vi "Sync AO and DO CTRdriven.vi"() -> ()   [LabVIEW 2021]
doc: "I. Description:\nThis example demonstrates how to continuously acquire and generate data at the same time, synchronized with one another.\n\nII. Instructions for Running:\n1. Select the physical channel to correspond to where your signal is input on the DAQ device. Also, select the corresponding channel for where your signal is being generated.\n2. Enter the minimum and maximum voltage ranges.\nNote: For better accuracy try to match the input range to the expected voltage level of the measured signal.\n3. Set the sample rate of the acquisition.\nNote: The rate should be at least twice as fast as the maximum frequency component of the signal being acquired. \n6. Select the Rate for the generation\n7. Select what type of signal to generate and the amplitude.\nNote: This example requires two DMA channels to run. If your hardware does not support two DMA channels, you need to set the Data Transfer Mechanism property for the Analog Output Task to use \"Interrupts\". The Data Transfer Mechanism property is located in the DAQmx Channel Property hierarchy at:\n\nDAQmx Channel Property Node>>Analog Output>>General Properties>>Advanced>>Data Transfer and Memory>>Data Transfer Mechanism\n\nRefer to your device documentation to determine how many DMA channels are supported for your hardware.\n\nIII. Block Diagram Steps:\n1. Create an analog input voltage channel. Also, create an analog output voltage channel.\n2. Set the rate for the sample clock. Additionally, define the sample mode to be continuous. Also, set the sample clock rate for the signal generation.\n2a. Call the Get Terminal Name with Device Prefix VI. This will take a Task and a terminal and create a properly formatted device + terminal name to use as the source of the Trigger.\n3. Define the parameters for a Digital Edge Start Trigger. Set the Analog output to trigger off the AI Start Trigger. This is an internal trigger signal.\n4. Use the Basic Function Generator VI to create the signal to be generated.\n5. Call the Start VI to arm the two functions. Make sure the analog output is armed before the analog input. This will ensure both will start at the same time.\n6. Read the waveform data in a loop until the user hits the stop button or an error occurs. The Is Task Done? VI is used to check for errors in the Analog Output Task.\n7. Call the Clear VI to Clear the Task\n8. Use the popup dialog box to display an error if any.\n\nIV. I/O Connections Overview:\nMake sure your signal input/output terminals match the Physical Channel I/O controls."
uses:
  <vilib>/Utility/error.llb/DialogType.ctl
  <vilib>/DAQmx/write.llb/DAQmx Write (Analog Wfm 1Chan NSamp).vi
  <vilib>/DAQmx/write.llb/DAQmx Write (Digital Wfm 1Chan NSamp).vi
  <vilib>/DAQmx/create/channels.llb/DAQmx Create Channel (DO-Digital Output).vi
  <vilib>/DAQmx/configure/timing.llb/DAQmx Timing (Sample Clock).vi
  <vilib>/DAQmx/create/channels.llb/DAQmx Create Channel (CO-Pulse Generation-Frequency).vi
  <vilib>/DAQmx/configure/timing.llb/DAQmx Timing (Implicit).vi
  <vilib>/DAQmx/create/channels.llb/DAQmx Create Channel (AO-Voltage-Basic).vi
  <vilib>/Waveform/DWDTOps.llb/Digital Pattern Generator (Ramp).vi
  <vilib>/Waveform/DWDTOps.llb/DWDT Uncompress Digital.vi
  <vilib>/DAQmx/miscellaneous.llb/DAQmx Fill In Error Info.vi
  <vilib>/Waveform/DWDTOps.llb/DWDT Digital Signal Subset.vi
  <vilib>/Waveform/DWDTOps.llb/DWDT Invert Digital.vi
  <resource>/objmgr/daqmx.rc
panel:
  out "Waveform Graph":dynamicdata(graph)
  out "Digital Waveform Graph":digitalwaveform(graph)
  out "Actual Update Generation Rate":dbl=5000.0 format="%0.2f"
  out "Actual Input Rate":dbl=10000.0 format="%0.2f"
  in  "rate":dbl=1000.0 caption="Analog Output Update Rate" format="%0.2f"
  in  "minimum value":dbl=-10.0 caption="Output Minimum Value" format="%0.2f"
  in  "maximum value":dbl=10.0 caption="Output Maximum Value" format="%0.2f"
  in  "physical channels":tag="Dev1/ao0" caption="Analog Output Physical Channel"
  in  "Physical Channel":tag="Dev1/port0/line0" caption="Digital Output Physical Channel"
  in  "Rate":dbl=1000.0 caption="Digital Output Update Rate" format="%0.2f"
  in  "stop":bool
  # "For instructions, select Help>>Show Context Help"
  # "Output Channel Parameters"
  # "Timing Parameters"
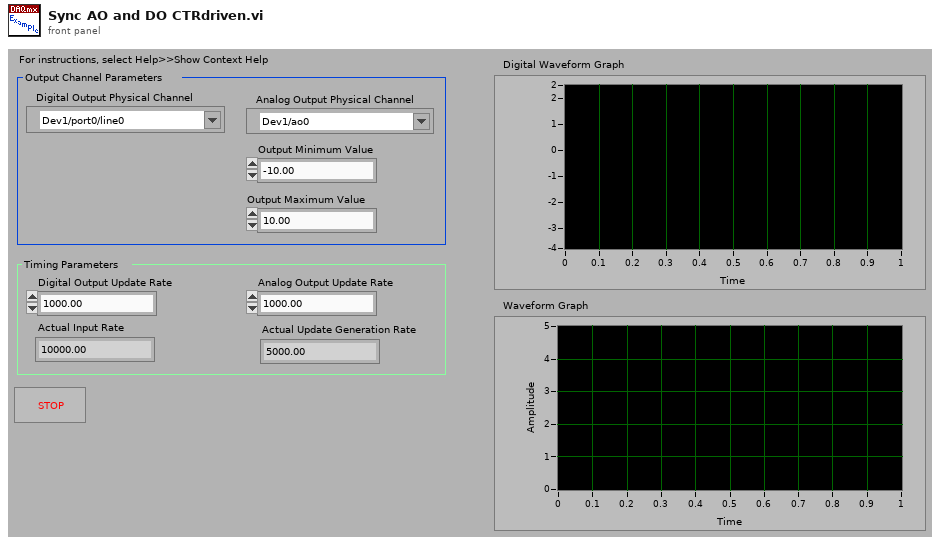
[diagram p1: front panel]
types:
  T1 = typedef "DialogType.ctl" = u16
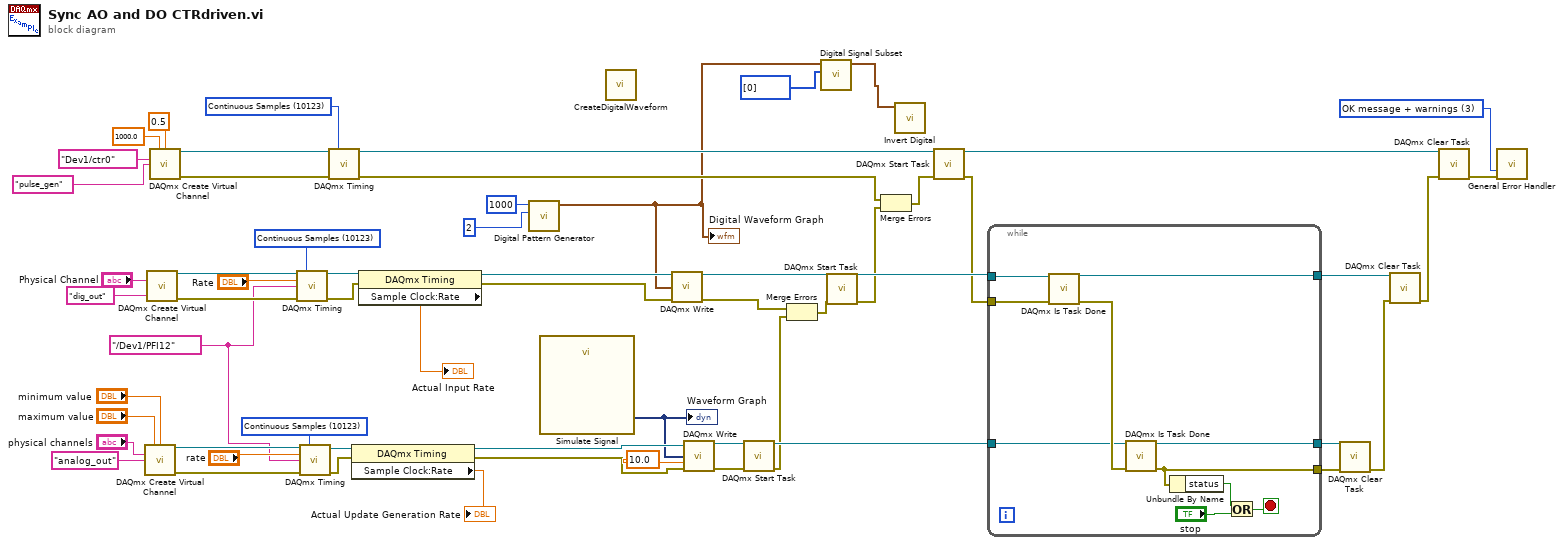
[diagram p0: block diagram]
diagram:
  w10 = 10123 items=["Finite Samples"=10178, "Continuous Samples"=10123, "Hardware Timed Single Point"=12522] ("sample mode")
  w6 = tag "/Dev1/PFI12" ("source")
  w43 = T1 3 items=["no dialog", "OK message", "continue or stop message", "OK message + warnings", "continue/stop + warnings"] ("type of dialog (OK msg:1)")
  w53 = 10123 items=["Finite Samples"=10178, "Continuous Samples"=10123] ("sample mode")
  w59 = 10123 items=["Finite Samples"=10178, "Continuous Samples"=10123] ("sample mode")
  n1 = call-poly <vilib>:"DAQmx Create Virtual Channel.vi"("maximum value"="maximum value", "minimum value"="minimum value", "physical channels"="physical channels", "name to assign"="analog_out") -> ("task out"=w52:refnum<k21>, "error out"=w51:errorcluster)  [unwired: 5 in, 5 out]
  n2 = call-poly <vilib>:"DAQmx Create Virtual Channel.vi"("lines"="Physical Channel", "name to assign"="dig_out") -> ("task out"=w57:refnum<k21>, "error out"=w58:errorcluster)  [unwired: 5 in, 7 out]
  n3 = call-poly <vilib>:"DAQmx Create Virtual Channel.vi"("frequency"=1000.0 ("High Time"), "duty cycle"=0.5 ("Low Time"), "counter"=tag "Dev1/ctr0" ("Counter(s)"), "name to assign"="pulse_gen") -> ("task out"=w12:refnum<k21>, "error out"=w11:errorcluster)  [unwired: 5 in, 5 out]
  n4 = call-poly <vilib>:"DAQmx Timing.vi"("task/channels in"=w57, "sample mode"=w59, "rate"="Rate", "source"=w6, "error in"=w58) -> ("task out"=w33:refnum<k21>, "error out"=w32:errorcluster)  [unwired: 2 in, 7 out]
  n5 = call-poly <vilib>:"DAQmx Timing.vi"("task/channels in"=w52, "sample mode"=w53, "rate"="rate", "source"=w6, "error in"=w51) -> ("task out"=w40:refnum<k21>, "error out"=w39:errorcluster)  [unwired: 2 in, 7 out]
  n6 = call-poly <vilib>:"DAQmx Timing.vi"("task/channels in"=w12, "sample mode"=w10, "error in"=w11) -> ("task out"=w9:refnum<k21>, "error out"=w8:errorcluster)  [unwired: 11 in]
  n7 = property class="DAQmx Timing"(reference=w40, error in=w39) -> (reference out=w41:refnum<k21>, error out=w38:errorcluster, "Sample Clock:Rate"=→"Actual Update Generation Rate":dbl)
  n8 = property class="DAQmx Timing"(reference=w33, error in=w32) -> (reference out=w28:refnum<k21>, error out=w27:errorcluster, "Sample Clock:Rate"=→"Actual Input Rate":dbl)
  n9 = call-poly <vilib>:"Digital Pattern Generator.vi"("number of signals"=u32 2, "number of samples"=u32 1000) -> ("digital waveform"=w1:digitalwaveform)  [unwired: 8 in, 1 out]
  "Digital Waveform Graph" <- w1
  n10 = call "Simulate Signal"() -> ("Triangle"=w24:dynamicdata)  [unwired: 6 in, 9 out]
  "Waveform Graph" <- w24
  n11 = call "CreateDigitalWaveform.vi"() -> ()  [unwired: 1 out]
  n12 = call-poly <vilib>:"DAQmx Write.vi"("task/channels in"=w28, "data"=w1, "error in"=w27) -> ("task out"=w25:refnum<k21>, "error out"=w26:errorcluster)  [unwired: 2 in, 9 out]
  n13 = call-poly <vilib>:"DAQmx Write.vi"("task/channels in"=w41, "data"=w24, "timeout"=10.0 ("Wirite Timeout"), "error in"=w38) -> ("task out"=w46:refnum<k21>, "error out"=w45:errorcluster)  [unwired: 1 in, 9 out]
  n14 = call <vilib>:"DAQmx Start Task.vi"("task/channels in"=w46, "error in"=w45) -> ("task out"=w50:refnum<k21>, "error out"=w36:errorcluster)  [unwired: 12 out]
  n15 = Merge Errors(w26, w36) -> (w35:errorcluster)
  n16 = call-poly <vilib>:"Digital Signal Subset.vi"("signals"=i32[] [0], "digital waveform"=w1) -> ("digital subset"=w2:digitalwaveform)  [unwired: 8 in, 1 out]
  n17 = call <vilib>:"DAQmx Start Task.vi"("task/channels in"=w25, "error in"=w35) -> ("task out"=w37:refnum<k21>, "error out"=w20:errorcluster)  [unwired: 12 out]
  n18 = Merge Errors(w8, w20) -> (w19:errorcluster)
  n19 = call-poly <vilib>:"Invert Digital.vi"("digital waveform"=w2) -> ()  [unwired: 9 in, 2 out]
  n20 = call <vilib>:"DAQmx Start Task.vi"("task/channels in"=w9, "error in"=w19) -> ("task out"=w17:refnum<k21>, "error out"=w18:errorcluster)  [unwired: 12 out]
  n21 = while {
    tunnel: [w70] -> w60
    tunnel: w50 -> [w65]
    tunnel: [w64] -> w49
    tunnel: w37 -> [w63]
    tunnel: w18 -> [w62]
    tunnel: [w61] -> w30
    stop <- w69 stop-if-true
    n22 = call <vilib>:"DAQmx Is Task Done.vi"("task/channels in"=w63, "error in"=w62) -> ("task out"=w70:refnum<k21>, "error out"=w66:errorcluster)  [unwired: 2 in, 10 out]
    n23 = call <vilib>:"DAQmx Is Task Done.vi"("task/channels in"=w65, "error in"=w66) -> ("task out"=w64:refnum<k21>, "error out"=w61:errorcluster)  [unwired: 12 out]
    n24 = Unbundle By Name(w61) -> ("status"=w67:bool)
    n25 = Or(x=w67, y="stop") -> (x .or. y?=w69:bool)
  }
  n26 = call <vilib>:"DAQmx Clear Task.vi"("task in"=w49, "error in"=w30) -> ("error out"=w29:errorcluster)  [unwired: 13 out]
  n27 = call <vilib>:"DAQmx Clear Task.vi"("task in"=w60, "error in"=w29) -> ("error out"=w16:errorcluster)  [unwired: 13 out]
  n28 = call <vilib>:"DAQmx Clear Task.vi"("task in"=w17, "error in"=w16) -> ("error out"=w15:errorcluster)  [unwired: 13 out]
  n29 = call <vilib>:"General Error Handler.vi"("type of dialog (OK msg:1)"=w43, "error in (no error)"=w15) -> ()  [unwired: 1 in, 13 out]
